vi "Close Panel.vi"(8 "error in (no error)":errorcluster, 10 "Close Panel":bool, 11 "Settings Model in":refnum<class "Settings Model.lvclass">) -> (0 "error out":errorcluster, 3 "Settings Model out":refnum<class "Settings Model.lvclass">)   [LabVIEW 2015, in "Settings Model.lvlib" / "Settings Model.lvclass"]
uses:
  Settings Model.lvclass
  <vilib>/ActorFramework/Actor/Actor.lvclass/Actor.ctl
  Settings Model.lvclass/Settings Model.ctl
  <vilib>/ActorFramework/Message Enqueuer/Message Enqueuer.lvclass/Message Enqueuer.ctl
  UI Controller/UI Controller Messages/Stop UI Msg/Stop UI Msg.lvclass
  <vilib>/Utility/miscctls.llb/LVPositionTypeDef.ctl
  UI Controller/UI Controller Messages/Hide Subpanel Msg/Hide Subpanel Msg.lvclass
  UI Controller/UI Controller Messages/Hide Subpanel Msg/Hide Subpanel Msg.lvclass/Hide Subpanel Msg.ctl
  <vilib>/ActorFramework/Self-Addressed Msg/Self-Addressed Msg.lvclass/Self-Addressed Msg.ctl
  <vilib>/ActorFrameworkMVC/View Controller/View Controller Messages/Insert Subpanel Msg/Insert Subpanel Msg.lvclass/Insert Subpanel Msg.ctl
  <vilib>/ActorFrameworkMVC/View Controller/View Controller Messages/Move Subpanel Msg/Move Subpanel Msg.lvclass/Move Subpanel Msg.ctl
  <vilib>/ActorFramework/Message Enqueuer/Enqueue.vi
  <vilib>/ActorFramework/Message Priority Queue/Priority Enqueue.vi
  <vilib>/ActorFramework/Self-Addressed Msg/Self-Addressed Msg.lvclass
  <vilib>/ActorFrameworkMVC/View Controller/View Controller Messages/Insert Subpanel Msg/Insert Subpanel Msg.lvclass
  <vilib>/ActorFrameworkMVC/View Controller/View Controller Messages/Move Subpanel Msg/Move Subpanel Msg.lvclass
  <vilib>/ActorFramework/Actor/Actor.lvclass
panel:
  # "NOTICE -- YOU MUST LEAVE THIS NOTICE IN PLACE.\n\nCopyright (c) 2015, LIANG LIU Shawn.Liu.cn@gmail.com\nAll rights reserved.\n\nRedistribution and use in source and binary forms, with or without modification, are permitted provided that the following conditions are met:\n-Redistributions of source code must retain the above copyright notice, this list of conditions and the following disclaimer.\n-Redistributions in binary form must reproduce the above copyright notice, this list of conditions and the following disclaimer in the documentation and/or other materials provided with the distribution.\n-Neither the name of the eLp nor the names of its contributors may be used to endorse or promote products derived from this software without specific prior written permission.\n\nTHIS SOFTWARE IS PROVIDED BY THE COPYRIGHT HOLDERS AND CONTRIBUTORS \"AS IS\" AND ANY EXPRESS OR IMPLIED WARRANTIES, INCLUDING, BUT NOT LIMITED TO, THE IMPLIED WARRANTIES OF MERCHANTABILITY AND FITNESS FOR A PARTICULAR PURPOSE ARE DISCLAIMED. IN NO EVENT SHALL THE COPYRIGHT HOLDER OR CONTRIBUTORS BE LIABLE FOR ANY DIRECT, INDIRECT, INCIDENTAL, SPECIAL, EXEMPLARY, OR CONSEQUENTIAL DAMAGES (INCLUDING, BUT NOT LIMITED TO, PROCUREMENT OF SUBSTITUTE GOODS OR SERVICES; LOSS OF USE, DATA, OR PROFITS; OR BUSINESS INTERRUPTION) HOWEVER CAUSED AND ON ANY THEORY OF LIABILITY, WHETHER IN CONTRACT, STRICT LIABILITY, OR TORT (INCLUDING NEGLIGENCE OR OTHERWISE) ARISING IN ANY WAY OUT OF THE USE OF THIS SOFTWARE, EVEN IF ADVISED OF THE POSSIBILITY OF SUCH DAMAGE."
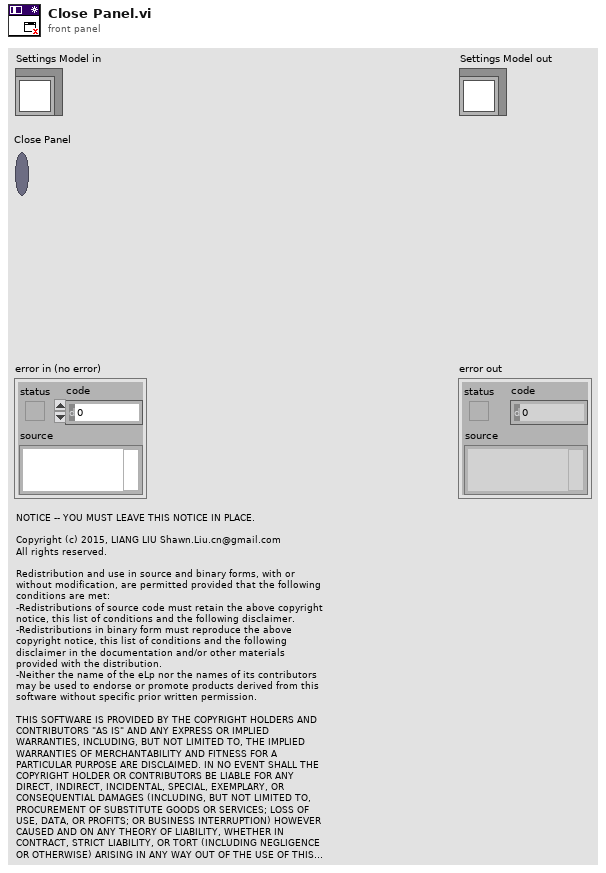
[diagram p1: front panel]
types:
  T1 = typedef "LVPositionTypeDef.ctl" = cluster{"Left":i32, "Top":i32}
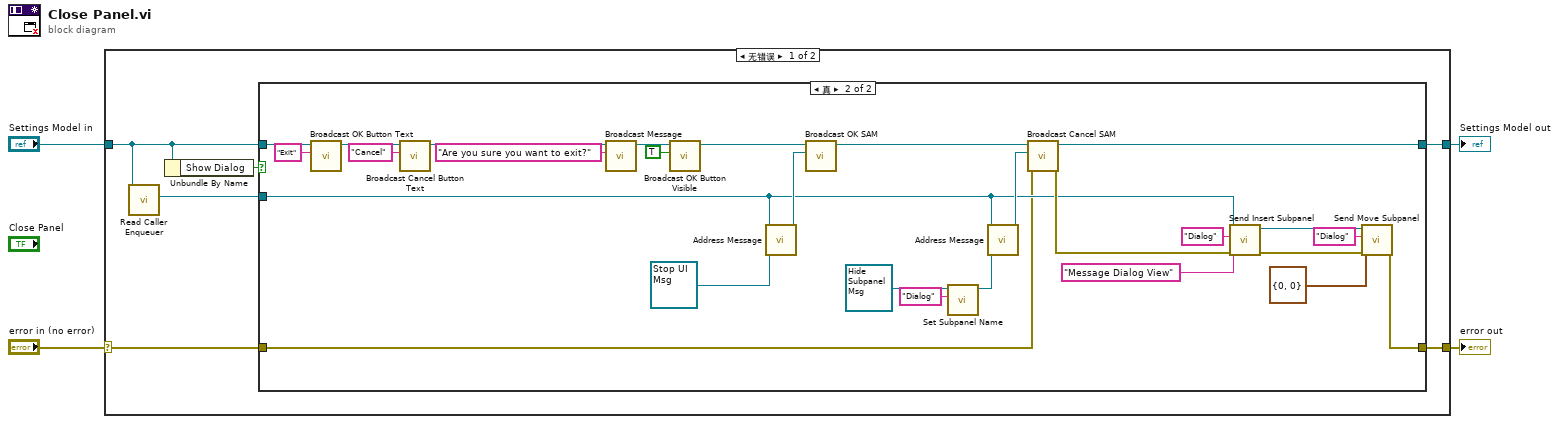
[diagram p0: block diagram]
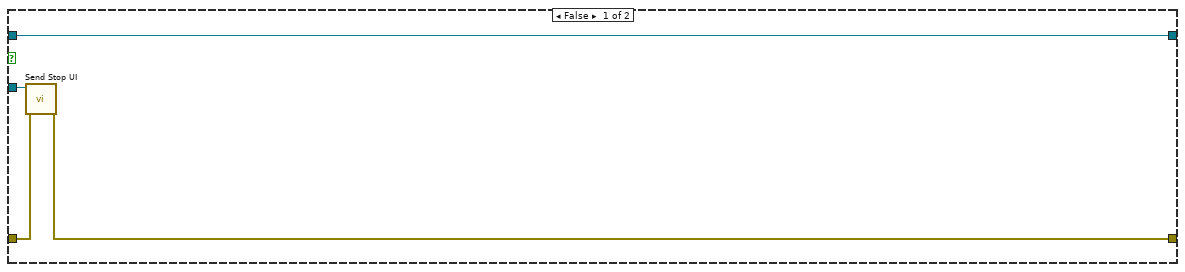
[diagram p2: hidden frame]
diagram:
  n1 = case shown="无错误" "error in (no error)" {
    selector: "error in (no error)" -> [w6 w43]
    tunnel: [w9 w42] -> w4
    tunnel: "Settings Model in" -> [w8 w42]
    tunnel: [w5 w43] -> w1
    frame No Error {
      n2 = call <vilib>:"Read Caller Enqueuer.vi"("Actor"=w8) -> ("Caller Enqueuer"=w7:refnum<class "Message Enqueuer.lvclass">)  [unwired: 10 in]
      n3 = Unbundle By Name(w8) -> ("Show Dialog"=w10:bool)
      n4 = case shown="真" w10 {
        tunnel: w8 -> [w14 w41]
        tunnel: [w14 w33] -> w9
        tunnel: w7 -> [w13 w25]
        tunnel: w6 -> [w12 w19]
        tunnel: [w11 w18] -> w5
        frame False {
          n5 = call "Send Stop UI.vi"("error in (no error)"=w12, "Message Enqueuer"=w13) -> ("error out"=w11:errorcluster)  [unwired: 8 in, 1 out]
        }
        frame True {
          n6 = call "Broadcast OK Button Text.vi"("OK Button Text"="Exit", "Settings Model in"=w41) -> ("Settings Model out"=w40:refnum<class "Settings Model.lvclass">)  [unwired: 8 in, 1 out]
          n7 = call "Broadcast Cancel Button Text.vi"("Cancel Button Text"="Cancel", "Settings Model in"=w40) -> ("Settings Model out"=w38:refnum<class "Settings Model.lvclass">)  [unwired: 8 in, 1 out]
          n8 = call "Broadcast Message.vi"("Message"="Are you sure you want to exit?", "Settings Model in"=w38) -> ("Settings Model out"=w36:refnum<class "Settings Model.lvclass">)  [unwired: 8 in, 1 out]
          n9 = call "Broadcast OK Button Visible.vi"("OK Button Visible"=TRUE, "Settings Model in"=w36) -> ("Settings Model out"=w21:refnum<class "Settings Model.lvclass">)  [unwired: 8 in, 1 out]
          n10 = call <vilib>:"Address Message.vi"("Message"=refnum<class "Stop UI Msg.lvclass"> refnum ("UI Controller.lvlib:Stop UI Msg.lvclass"), "Destination"=w25) -> ("Self-Addressed Message"=w31:refnum<class "Self-Addressed Msg.lvclass">)  [unwired: 9 in]
          n11 = call "Broadcast OK SAM.vi"("OK SAM"=w31, "Settings Model in"=w21) -> ("Settings Model out"=w34:refnum<class "Settings Model.lvclass">)  [unwired: 8 in, 1 out]
          n12 = call "Set Subpanel Name.vi"("Subpanel Name"="Dialog", "Hide Subpanel Msg in"=refnum<class "Hide Subpanel Msg.lvclass"> refnum ("View Controller.lvlib:Move Subpanel Msg.lvclass")) -> ("Hide Subpanel Msg out"=w15:refnum<class "Hide Subpanel Msg.lvclass">)  [unwired: 9 in]
          n13 = call <vilib>:"Address Message.vi"("Message"=w15, "Destination"=w25) -> ("Self-Addressed Message"=w30:refnum<class "Self-Addressed Msg.lvclass">)  [unwired: 9 in]
          n14 = call "Broadcast Cancel SAM.vi"("error in (no error)"=w19, "Cancel SAM"=w30, "Settings Model in"=w34) -> ("error out"=w27:errorcluster, "Settings Model out"=w33:refnum<class "Settings Model.lvclass">)  [unwired: 7 in]
          n15 = call <vilib>:"Send Insert Subpanel.vi"("error in (no error)"=w27, "View Name"="Message Dialog View" ("Subpanel Name"), "Subpanel Name"="Dialog", "Message Enqueuer"=w25) -> ("error out"=w26:errorcluster, "Message Enqueuer out"=w24:refnum<class "Message Enqueuer.lvclass">)  [unwired: 6 in]
          n16 = call <vilib>:"Send Move Subpanel.vi"("error in (no error)"=w26, "Position"=T1 {"Left"=0, "Top"=0}, "Subpanel Name"="Dialog", "Message Enqueuer"=w24) -> ("error out"=w18:errorcluster)  [unwired: 6 in, 1 out]
        }
      }
    }
    frame Error {
    }
  }
  "error out" <- w1
  "Settings Model out" <- w4
